vi "Car Wash Timer.vi"(7 "Proximity switch":bool, 8 "error in (no error)":errorcluster, 10 "Time Target (s)":dbl, 11 "Command":T2) -> (0 "error out":errorcluster, 2 "Status":T1)   [LabVIEW 2013]
doc: "Feedback node implementation of the car wash timer"
uses:
  Type Defs/Car Wash Timer Enum.ctl
  Shared Files/Shared Type Defs/Cycle Status Cluster.ctl
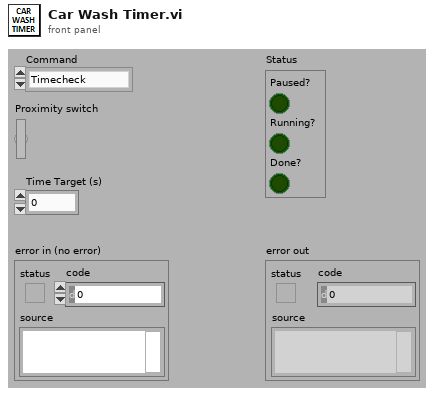
[diagram p1: front panel]
types:
  T1 = typedef "Cycle Status Cluster.ctl" = cluster{"Paused?":bool, "Running?":bool, "Done?":bool}
  T2 = typedef "Car Wash Timer Enum.ctl" = enum16{"Timecheck", "Reset"}
  T3 = cluster{"Last Time Stamp":dbl, "Elapsed Time (s)":dbl}
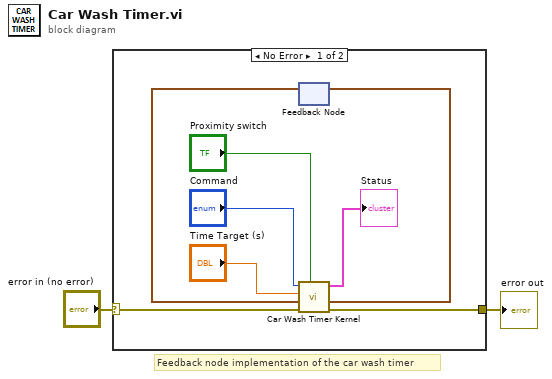
[diagram p0: block diagram]
diagram:
  # "Feedback node implementation of the car wash timer"
  n1 = case shown="No Error" "error in (no error)" {
    selector: "error in (no error)" -> [w6 w11]
    tunnel: [w5 w11] -> w1
    frame No Error {
      n2 = feedback #1() -> (w3:T3)  [unwired: 1 in]
      n3 = call "Car Wash Timer Kernel.vi"("Proximity switch"="Proximity switch", "error in (no error)"=w6, "Timer Data in"=w3, "Time Target (s)"="Time Target (s)", "Command"="Command") -> ("error out"=w5:errorcluster, "Timer Data out"=w4:T3, "Status"=→"Status":T1)  [unwired: 4 in]
      n4 = feedback-in #1(w4) -> ()
    }
    frame Error {
    }
  }
  "error out" <- w1
